vi "Pre-Build VI - Run Unit Tests.vi"(8 "error in (no error)":errorcluster) -> (0 "error out":errorcluster, 1 "VIs without test coverage":string[](array[string]), 2 "error type":enum16{"fatal", "non-fatal", "warning"}(ring), 4 "VIs not loadable":string[](array[string]), 5 "Failed Tests":string[](array[string]))   [LabVIEW 2009]
uses:
  <userlib>/_OpenG.lib/array/array.llb/Conditional Auto-Indexing Tunnel (String)__ogtk.vi
  <userlib>/_OpenG.lib/array/array.llb/Empty 1D Array (String)__ogtk.vi
  <userlib>/_OpenG.lib/array/array.llb/Filter 1D Array (String)__ogtk.vi
panel:
  in  "type specifier VI Refnum (for type only)":refnum<vi>
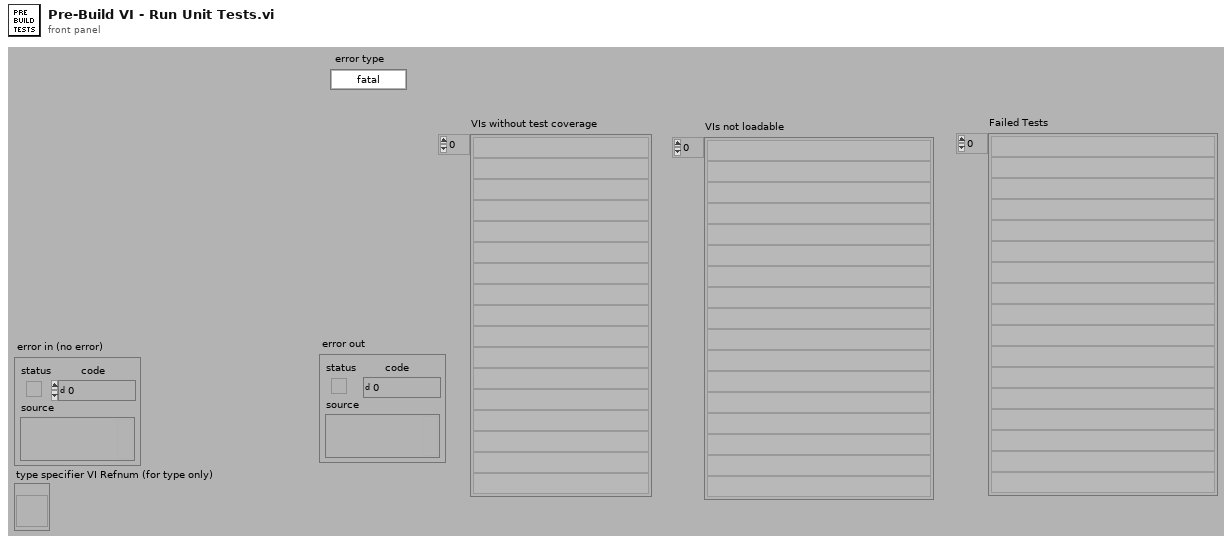
[diagram p1: front panel]
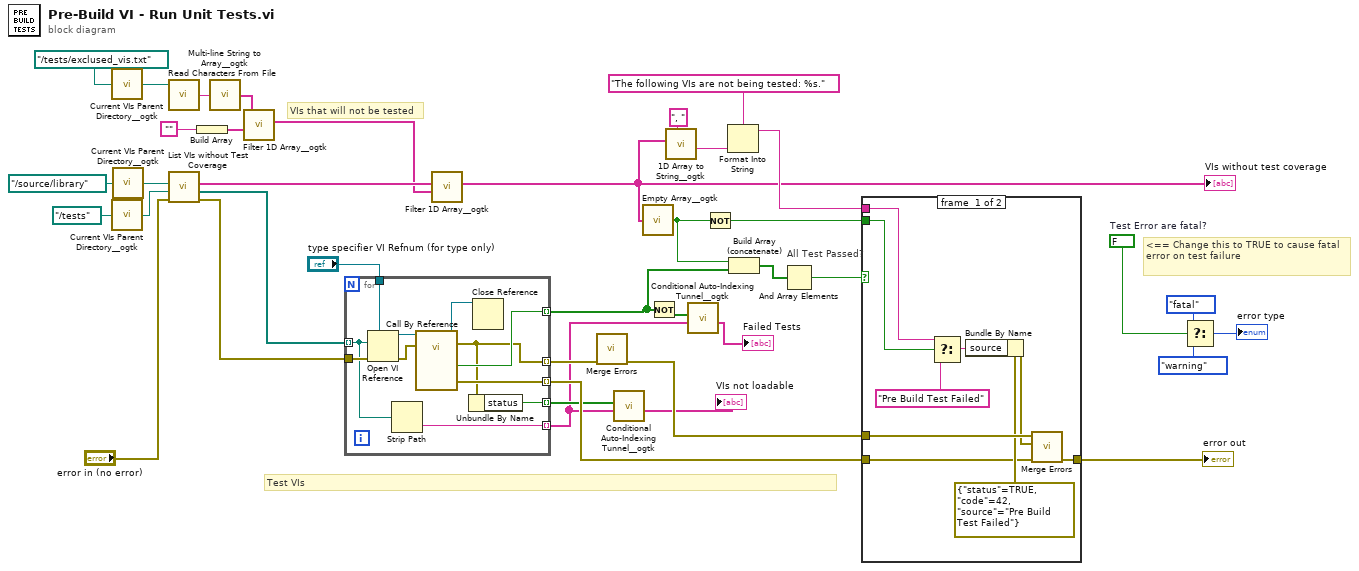
[diagram p0: block diagram]
diagram:
  w26 = FALSE  # Test Error are fatal?
  # "VIs that will not be tested"
  # "<== Change this to TRUE to cause fatal error on test failure"
  # "All Test Passed?"
  # "Test VIs"
  n1 = call <userlib>:"Current VIs Parent Directory__ogtk.vi"("Relative path (.)"=path "../tests/exclused_vis.txt") -> ("Parent Directory (+ Relative)"=w16:path)  [unwired: 4 in]
  n2 = call <userlib>:"Current VIs Parent Directory__ogtk.vi"("Relative path (.)"=path "../tests") -> ("Parent Directory (+ Relative)"=w21:path)  [unwired: 4 in]
  n3 = call <userlib>:"Current VIs Parent Directory__ogtk.vi"("Relative path (.)"=path "../source/library") -> ("Parent Directory (+ Relative)"=w30:path)  [unwired: 4 in]
  n4 = call <vilib>:"Read Characters From File.vi"("file path (dialog if empty)"=w16) -> ("character string"=w15:string)  [unwired: 5 in, 3 out]
  n5 = call "List VIs without Test Coverage.vi"("error in (no error)"="error in (no error)", "Tests Root"=w21, "Source Root"=w30) -> ("error out"=w10:errorcluster, "Test VIs"=w20:path[], "VIs without test coverage"=w37:string[])  [unwired: 6 in]
  n6 = Build Array("") -> (w12:string[])
  n7 = call <userlib>:"Multi-line String to Array__ogtk.vi"("string"=w15) -> ("lines"=w14:string[])
  n8 = call-poly <userlib>:"Filter 1D Array__ogtk.vi"("items to filter"=w12, "array"=w14) -> ("filtered array"=w11:string[])  [unwired: 4 in, 1 out]
  n9 = for {
    tunnel: w20 -> [w41] mode=indexing
    tunnel: "type specifier VI Refnum (for type only)" -> [w50]
    tunnel: [w47] -> w5 mode=indexing
    tunnel: [w45] -> w18 mode=indexing
    tunnel: w10 -> [w44]
    tunnel: [w43] -> w8 mode=indexing
    tunnel: [w42] -> w7 mode=indexing
    tunnel: [w40] -> w3 mode=indexing
    n10 = Open VI Reference(type specifier VI Refnum (for type only)=w50, vi path=w41, error in (no error)=w44) -> (vi reference=w49:refnum<vi>, error out=w48:errorcluster)  [unwired: 3 in]
    n11 = Strip Path(path=w41) -> (name=w40:string)  [unwired: 1 out]
    n12 = call-by-ref "?"(reference=w49, error in=w48) -> (reference out=w46:refnum<vi>, error out=w43:errorcluster, 0:"error out"=w45:errorcluster, "pass"=w47:bool)  [unwired: 10 in]
    n13 = Unbundle By Name(w43) -> ("status"=w42:bool)
    n14 = Close Reference(reference=w46) -> ()  [unwired: 1 in, 1 out]
  }
  n15 = call-poly <userlib>:"Filter 1D Array__ogtk.vi"("items to filter"=w11, "array"=w37) -> ("filtered array"=w1:string[])  [unwired: 4 in, 1 out]
  "VIs without test coverage" <- w1
  n16 = call <vilib>:"Merge Errors.vi"("error array in"=w8) -> ("error out"=w9:errorcluster)  [unwired: 6 in]
  n17 = call-poly <userlib>:"Conditional Auto-Indexing Tunnel__ogtk.vi"("Array in"=w3, "Elements to keep"=w7) -> ("Filtered Array out"=→"VIs not loadable":string[])  [unwired: 5 in]
  n18 = call-poly <userlib>:"Empty Array__ogtk.vi"("Array"=w1) -> ("Empty Array?"=w32:bool)  [unwired: 8 in]
  n19 = Not(x=w5) -> (.not. x?=w4:bool[])
  n20 = call <userlib>:"1D Array to String__ogtk.vi"("delimiter (Tab)"=", ", "Array of Strings"=w1) -> ("delimited string"=w35:string)  [unwired: 9 in]
  n21 = call-poly <userlib>:"Conditional Auto-Indexing Tunnel__ogtk.vi"("Array in"=w3, "Elements to keep"=w4) -> ("Filtered Array out"=→"Failed Tests":string[])  [unwired: 5 in]
  n22 = Not(x=w32) -> (.not. x?=w31:bool)
  n23 = Format Into String(format string="The following VIs are not being tested: %s.", w35) -> (resulting string=w33:string)  [unwired: 2 in, 1 out]
  n24 = Build Array (concatenate)(w32, w5) -> (w39:bool[])
  n25 = And Array Elements(Boolean array=w39) -> (logical AND=w38:bool)
  n26 = case shown="False" w38 {
    tunnel: w9 -> [w59 w60]
    tunnel: [w58 w60] -> w28
    tunnel: w31 -> [w57 _]
    tunnel: w33 -> [w56 _]
    tunnel: w18 -> [w51 _]
    frame #0 {
      n27 = Select(t=w56, s=w57, f="Pre Build Test Failed" ("source")) -> (s? t:f=w54:string)
      n28 = Bundle By Name(cluster=errorcluster {"status"=TRUE, "code"=42, "source"="Pre Build Test Failed"} ("error out"), "source"=w54) -> (w53:errorcluster)
      n29 = call <vilib>:"Merge Errors.vi"("error array in"=w51, "error in 2 (no error)"=w53, "error in 1 (no error)"=w59) -> ("error out"=w58:errorcluster)  [unwired: 4 in]
    }
    frame #1 {
    }
  }
  "error out" <- w28
  n30 = Select(t=enum16{"fatal", "non-fatal", "warning"}."fatal" ("error type"), s=w26, f=enum16{"fatal", "non-fatal", "warning"}."warning" ("error type")) -> (s? t:f=→"error type":enum16{"fatal", "non-fatal", "warning"})
